vi "FilterAndReorderChannels.vi"(8 "error in (no error)":errorcluster, 10 "channels":T7[](array[typedef]), 11 "device":T1) -> (0 "error out":errorcluster, 2 "acquisition channels (in acquisition order)":T7[](array[typedef]))   [LabVIEW 2015]
uses:
  <vilib>/addons/InsightCM/MessageBus/Base/controls/Channel.ctl
  <vilib>/addons/InsightCM/MessageBus/Base/controls/KeyValuePair.ctl
  <vilib>/addons/InsightCM/MessageBus/Base/controls/MetricModel.ctl
  <vilib>/addons/InsightCM/MessageBus/Base/controls/Device.ctl
  <vilib>/addons/InsightCM/MessageBus/Base/controls/DataGroup.ctl
  <vilib>/addons/InsightCM/MessageBus/Base/controls/OperatingState.ctl
  <vilib>/addons/InsightCM/MessageBus/Base/controls/Trigger.ctl
  <vilib>/addons/InsightCM/MessageBus/Base/controls/Condition.ctl
  <vilib>/addons/InsightCM/Utilities/PropertyHelpers/PropertyHelpers.lvlib
panel:
  out "hardware channel name (in acquisition order)":string[](array[string])
  out "channel IDs (in acquisition order)":string[](array[string])
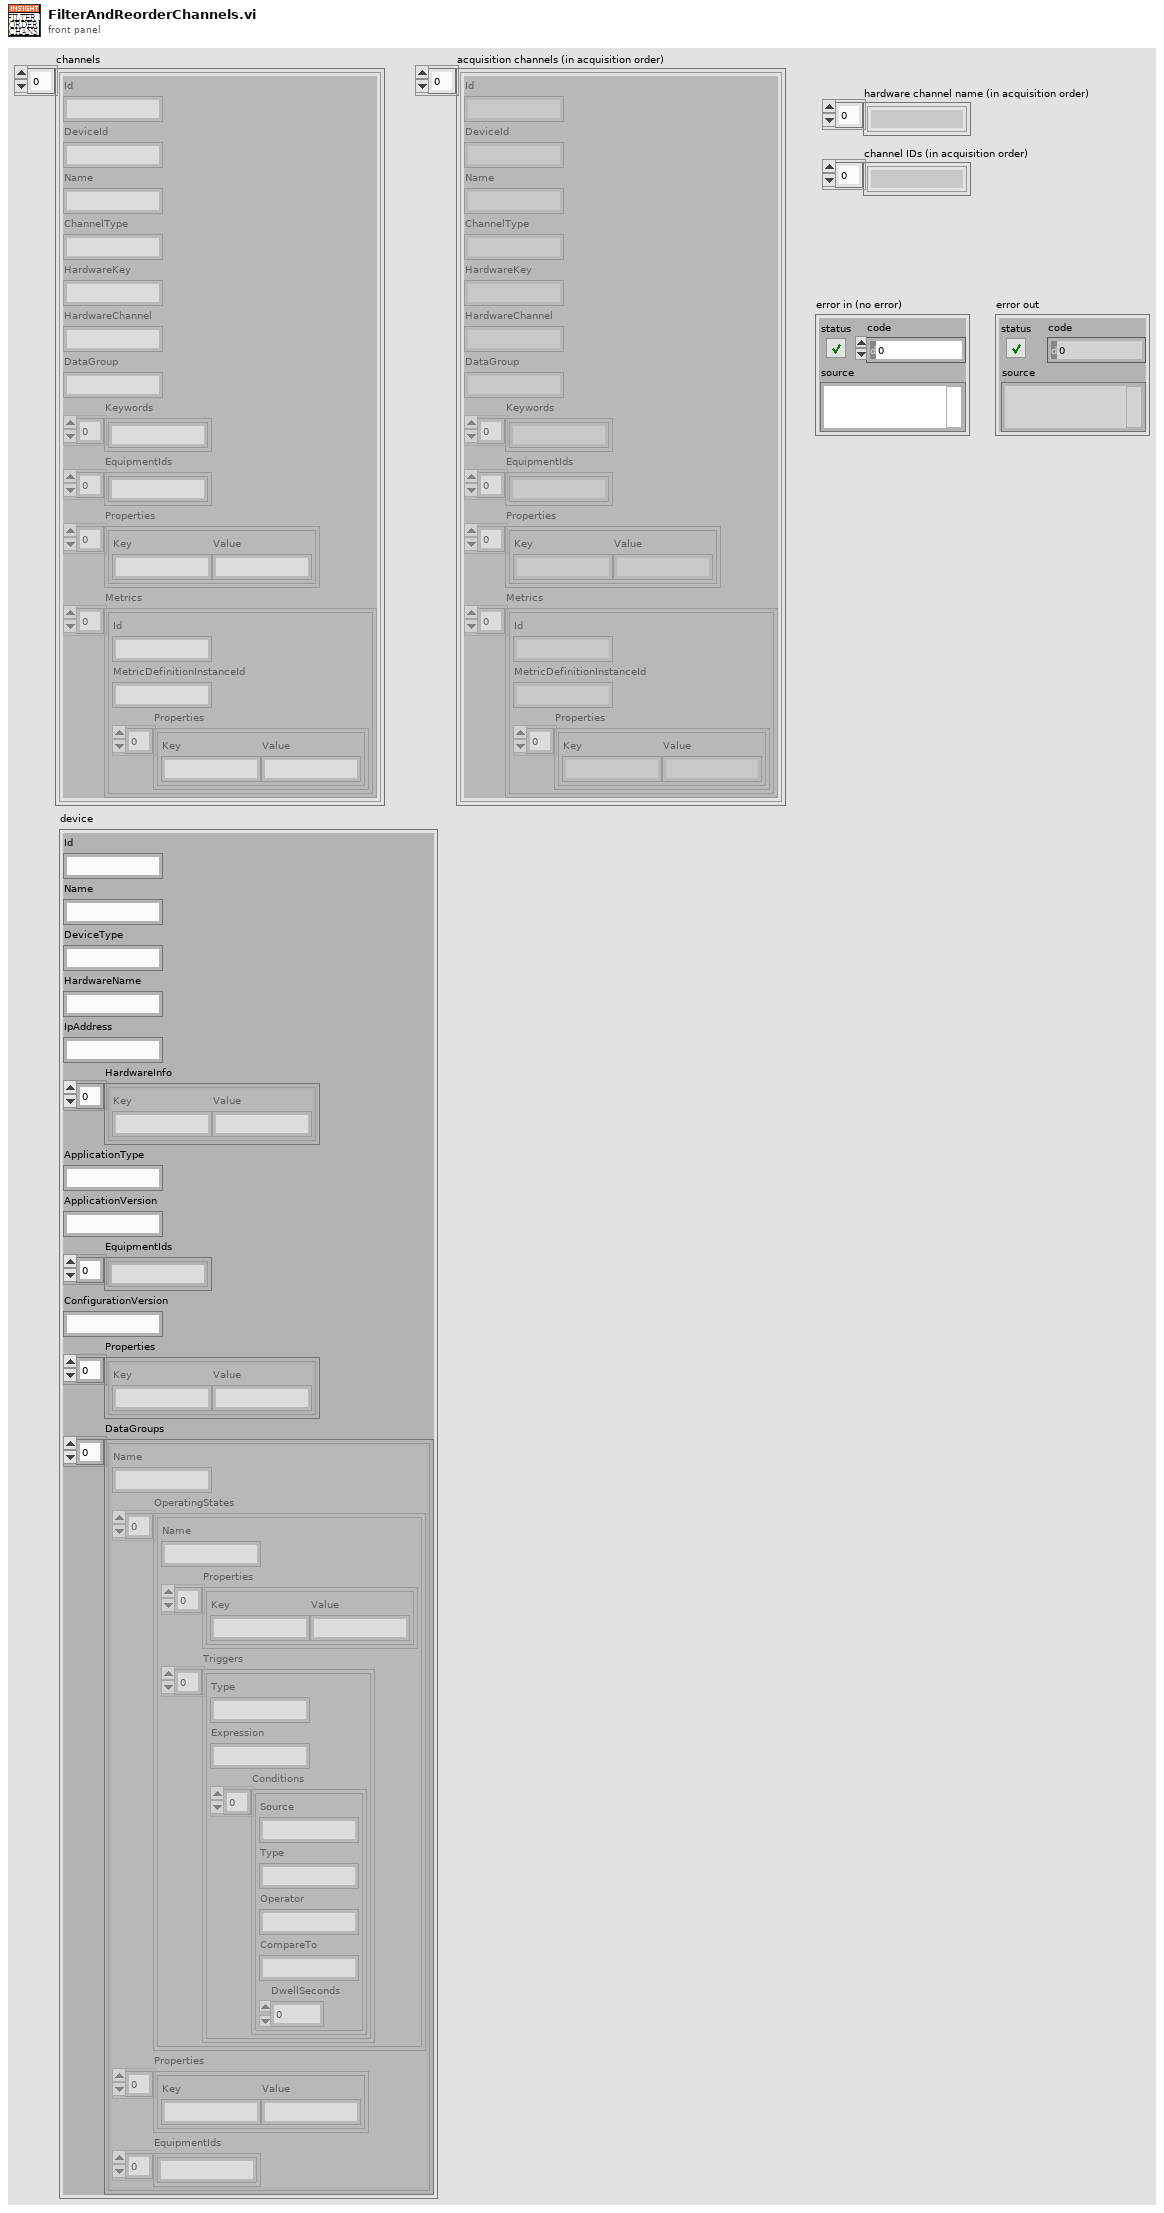
[diagram p1: front panel]
types:
  T1 = typedef "Device.ctl" = cluster{"Id":string, "Name":string, "DeviceType":string, "HardwareName":string, "IpAddress":string, "HardwareInfo":T2[], "ApplicationType":string, "ApplicationVersion":string, "EquipmentIds":string[], "ConfigurationVersion":string, "Properties":T2[], "DataGroups":T3[]}
  T2 = typedef "KeyValuePair.ctl" = cluster{"Key":string, "Value":string}
  T3 = typedef "DataGroup.ctl" = cluster{"Name":string, "OperatingStates":T4[], "Properties":T2[], "EquipmentIds":string[]}
  T4 = typedef "OperatingState.ctl" = cluster{"Name":string, "Properties":T2[], "Triggers":T5[]}
  T5 = typedef "Trigger.ctl" = cluster{"Type":string, "Expression":string, "Conditions":T6[]}
  T6 = typedef "Condition.ctl" = cluster{"Source":string, "Type":string, "Operator":string, "CompareTo":string, "DwellSeconds":dbl}
  T7 = typedef "Channel.ctl" = cluster{"Id":string, "DeviceId":string, "Name":string, "ChannelType":string, "HardwareKey":string, "HardwareChannel":string, "DataGroup":string, "Keywords":string[], "EquipmentIds":string[], "Properties":T2[], "Metrics":T8[]}
  T8 = typedef "MetricModel.ctl" = cluster{"Id":string, "MetricDefinitionInstanceId":string, "Properties":T2[]}
  T9 = cluster{"HardwareChannel":string, "Id":string, "ChannelModel":T7}
  T10 = cluster{"HardwareChannel":string, "Id":string, "ChannelModel":T7}[]
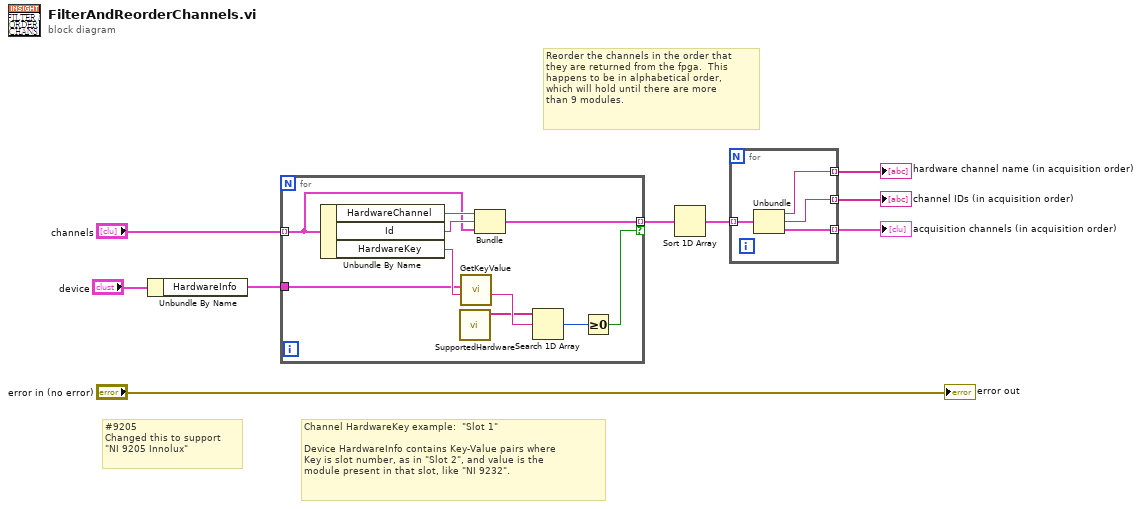
[diagram p0: block diagram]
diagram:
  # "#9205\nChanged this to support\n\"NI 9205 Innolux\""
  # "Channel HardwareKey example:  \"Slot 1\"\n\nDevice HardwareInfo contains Key-Value pairs where\nKey is slot number, as in \"Slot 2\", and value is the\nmodule present in that slot, like \"NI 9232\"."
  # "Reorder the channels in the order that\nthey are returned from the fpga.  This\nhappens to be in alphabetical order,\nwhich will hold until there are more\nthan 9 modules."
  n1 = Unbundle By Name("device") -> ("HardwareInfo"=w1:T2[])
  n2 = for {
    tunnel: "channels" -> [w16] mode=indexing
    tunnel: [w18] -> w5 mode=indexing if=w14
    tunnel: w1 -> [w11]
    n3 = Unbundle By Name(w16) -> ("HardwareChannel"=w19:string, "Id"=w17:string, "HardwareKey"=w12:string)
    n4 = call "SupportedHardware.vi"() -> ("Supported Hardware"=w10:string[])  [unwired: 11 in]
    n5 = call <vilib>:"GetKeyValue.vi"("key"=w12, "key value pairs"=w11) -> ("value"=w13:string)  [unwired: 7 in, 2 out]
    n6 = Bundle("HardwareChannel"=w19, "Id"=w17, "ChannelModel"=w16) -> (w18:T9)  [unwired: 1 in]
    n7 = Search 1D Array(1D array=w10, element=w13) -> (index of element=w15:i32)  [unwired: 1 in]
    n8 = Greater Or Equal To 0?(x=w15) -> (x >= 0?=w14:bool)
  }
  n9 = Sort 1D Array(array=w5) -> (sorted array=w6:T10)
  n10 = for {
    tunnel: w6 -> [w23] mode=indexing
    tunnel: [w22] -> w8 mode=indexing
    tunnel: [w21] -> w9 mode=indexing
    tunnel: [w20] -> w3 mode=indexing
    n11 = Unbundle(w23) -> ("HardwareChannel"=w20:string, "Id"=w22:string, "ChannelModel"=w21:T7)
  }
  "acquisition channels (in acquisition order)" <- w9
  "channel IDs (in acquisition order)" <- w8
  "hardware channel name (in acquisition order)" <- w3
  "error out" <- "error in (no error)"
